vi "Learn.vi"(8 "error in (no error)":errorcluster, 11 "VISA resource name":refnum<visa-resource-name>) -> (0 "error out":errorcluster, 2 "Query Response":string, 3 "VISA resource name out":refnum<visa-resource-name>)   [LabVIEW 2015, in "Agilent 428X Series.lvlib"]
doc: "The learn query tells the HP 4284A to send a response that contains all the necessary commands to set the HP 4284A to its present state. The response can later be sent back to the HP 4284A to place it in this state. This provides the user with a means of setting up a device manually and then reading the device setting and storing the information for later use."
uses:
  Agilent 428X Series.lvlib
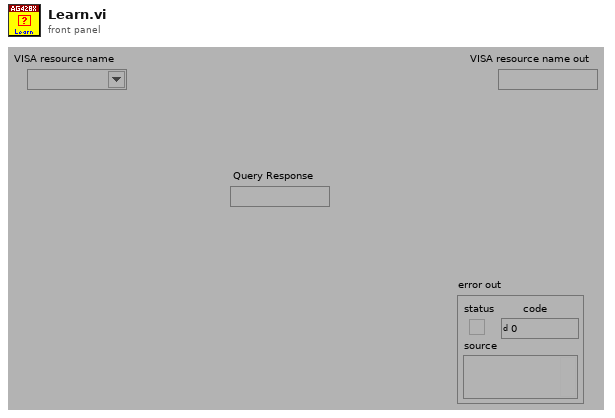
[diagram p1: front panel]
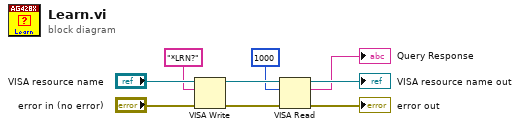
[diagram p0: block diagram]
diagram:
  n1 = VISA Write(VISA resource name="VISA resource name", write buffer="*LRN?" ("write buffer (\"\")"), error in (no error)="error in (no error)") -> (VISA resource name out=w8:refnum<visa-resource-name>, error out=w5:errorcluster)  [unwired: 1 out]
  n2 = VISA Read(VISA resource name=w8, byte count=u32 1000 ("byte count (0)"), error in (no error)=w5) -> (VISA resource name out=→"VISA resource name out":refnum<visa-resource-name>, read buffer=→"Query Response":string, error out=→"error out":errorcluster)  [unwired: 1 out]
